vi "roboRIO Event Create Once.vi"(7 "ini":bool) -> (3 "roboRIO Events":refnum<user-event>, 4 "Camera Events 2":T1={"Event Type"=enum."Exit", "AirTag Info Array"=[]})   [LabVIEW 2025]
uses:
  roboRIO Event Cluster.ctl
  roboRIO Event Setup Types.ctl
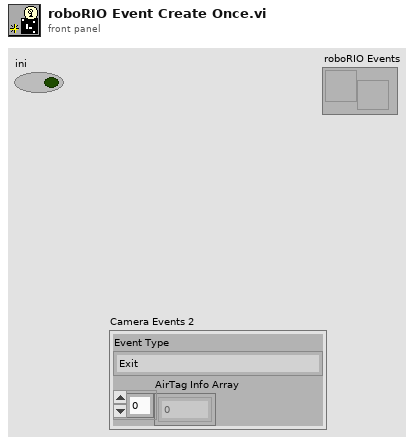
[diagram p1: front panel]
types:
  T1 = typedef "roboRIO Event Cluster.ctl" = cluster{"Event Type":T2, "AirTag Info Array":dbl[]}
  T2 = typedef "roboRIO Event Setup Types.ctl" = enum16{"Default", "Send Data", "Exit"}
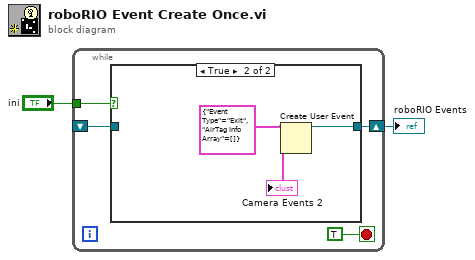
[diagram p0: block diagram]
diagram:
  n1 = while {
    shift-right: [w5] -> w1
    shift-left: _ -> [w4]
    tunnel: "ini" -> [w3]
    stop <- TRUE stop-if-true
    n2 = case shown="True" w3 {
      tunnel: [w7 w9] -> w5
      tunnel: w4 -> [w7 _]
      frame False {
      }
      frame True {
        w8 = T1 {"Event Type"=enum."Exit", "AirTag Info Array"=[]} ("roboRIO Events")
        n3 = Create User Event(user event datatype=w8) -> (user event=w9:refnum<user-event>)  [unwired: 1 in, 1 out]
        "Camera Events 2" <- w8
      }
    }
  }
  "roboRIO Events" <- w1
